vi "Logout Status Msg.vi"(10 "Logout":refnum<vi>, 11 "String in":refnum<vi>) -> ()   [LabVIEW 2019]
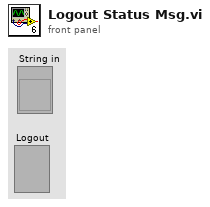
[diagram p1: front panel]
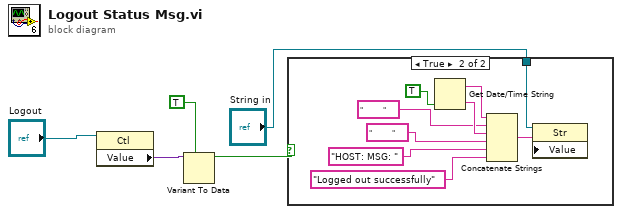
[diagram p0: block diagram]
diagram:
  n1 = property class="Ctl"(reference="Logout") -> ("Value"=w3:variant)  [unwired: 1 in, 2 out]
  n2 = Variant To Data(type=TRUE, Variant=w3) -> (data=w4:bool)  [unwired: 1 in, 1 out]
  n3 = case shown="True" w4 {
    tunnel: "String in" -> [_ w6]
    frame False {
    }
    frame True {
      n4 = Get Date/Time String(want seconds? (F)=TRUE) -> (date string=w12:string, time string=w13:string)  [unwired: 2 in]
      n5 = Concatenate Strings(w12, "          ", w13, "          ", "HOST: MSG: " ("string"), "Logged out successfully" ("String")) -> (w14:string)
      n6 = property class="Str"(reference=w6, "Value"=w14) -> ()  [unwired: 1 in, 2 out]
    }
  }
